vi "2Dto1D(SubVI).vi"(1 "X1":dbl[][](array[numeric])) -> (0 "Y1":dbl[](array[numeric]))   [LabVIEW 2017]
panel:
  # "2D 입력"
  # "1D 출력"
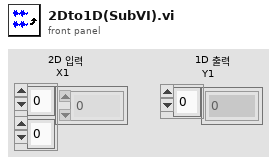
[diagram p1: front panel]
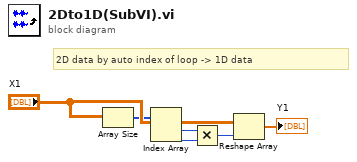
[diagram p0: block diagram]
diagram:
  # "2D data by auto index of loop -> 1D data"
  n1 = Array Size(array="X1") -> (size(s)=w5:i32[])
  n2 = Index Array(array=w5) -> (element #1=w3:i32, element #2=w4:i32)  [unwired: 2 in]
  n3 = Multiply(x=w3, y=w4) -> (x*y=w2:i32)
  n4 = Reshape Array("X1", w2) -> (→"Y1":dbl[])
